vi "Handle Error.vi"(8 "error in (no error)":errorcluster, 11 "Controller in":refnum<class "Controller.lvclass">) -> (0 "error out":errorcluster, 2 "stop actor?":bool=TRUE, 3 "Controller out":refnum<class "Controller.lvclass">)   [LabVIEW 2017, in "Controller Actor.lvlib" / "Controller.lvclass"]
doc: "(<B>Filename</B>: Actor Framework.lvlib:Actor.lvclass:Handle Error.vi)\n\nDefines how the actor handles an error that occurred while processing a message.\n\nBy default, this method does nothing except stop the actor. This method also treats error code 43 (coming from <B>error in</B>) as a sign that the actor shut down normally. In this situation, the Handle Error method does not return the error on <B>error out</B>, meaning the actor's caller will not receive it. All other error codes will be returned on <B>error out</B>.\n\nA descendant class may override this method to change this behavior."
uses:
  Controller.lvclass
  <vilib>/ActorFramework/Actor/Actor.lvclass
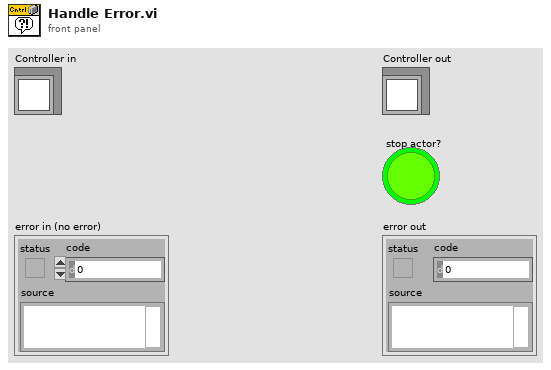
[diagram p1: front panel]
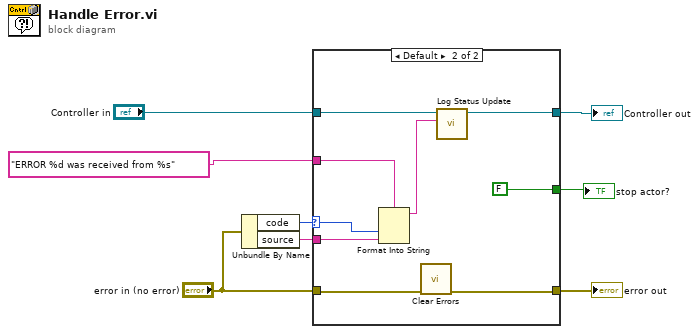
[diagram p0: block diagram]
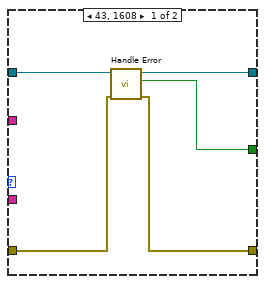
[diagram p2: hidden frame]
diagram:
  n1 = Unbundle By Name("error in (no error)") -> ("code"=w4:i32, "source"=w5:string)
  n2 = case shown="Default" w4 {
    selector: w4 -> [_ w16]
    tunnel: "Controller in" -> [w12 w22]
    tunnel: [w13 w21] -> w8
    tunnel: "error in (no error)" -> [w10 w20]
    tunnel: [w9 w19] -> w7
    tunnel: [w11 FALSE ("stop actor?")] -> w6
    tunnel: w5 -> [_ w17]
    tunnel: "ERROR %d was received from %s" ("format string") -> [_ w14]
    frame 43, 1608 {
      n3 = call-parent "Handle Error.vi"("error in (no error)"=w10, "Actor in"=w12) -> ("error out"=w9:errorcluster, "stop actor?"=w11:bool, "Actor out"=w13:refnum<class "Controller.lvclass">)  [unwired: 7 in]
    }
    frame Default {
      n4 = Format Into String(format string=w14, w16, w17) -> (resulting string=w15:string)  [unwired: 2 in, 1 out]
      n5 = call <vilib>:"Clear Errors.vi"("error in (no error)"=w20) -> ("error out"=w19:errorcluster)  [unwired: 5 in, 1 out]
      n6 = call-dynamic "Log Status Update.vi"("String"=w15, "Controller in"=w22) -> ("Controller out"=w21:refnum<class "Controller.lvclass">)  [unwired: 8 in, 1 out]
    }
  }
  "Controller out" <- w8
  "error out" <- w7
  "stop actor?" <- w6
